vi "Read Pin.vi"(8 "error in (no error)":errorcluster, 9 "Pin 2":dbl caption="Pin", 10 "Port 4":dbl caption="Port", 11 "Arduino in":refnum<class "Arduino.lvclass">) -> (0 "error out":errorcluster, 3 "Arduino out":refnum<class "Arduino.lvclass">)   [LabVIEW 2020, in "Arduino.lvclass"]
uses:
  Arduino.lvclass
  Arduino.lvclass/Arduino.ctl
  713354a0-7d03-489a-938a-0a5a614069ab.vi
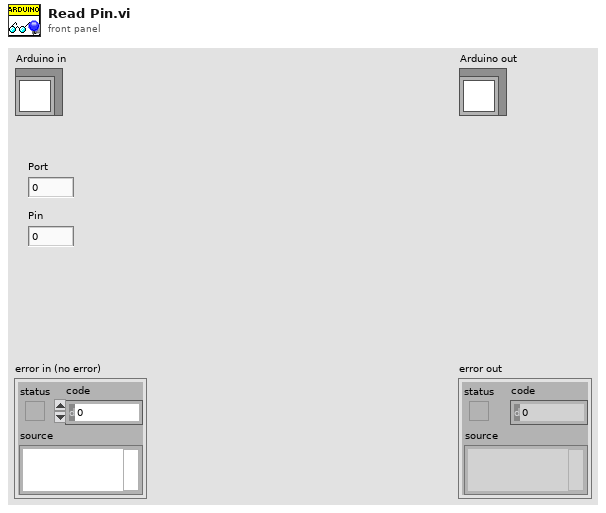
[diagram p1: front panel]
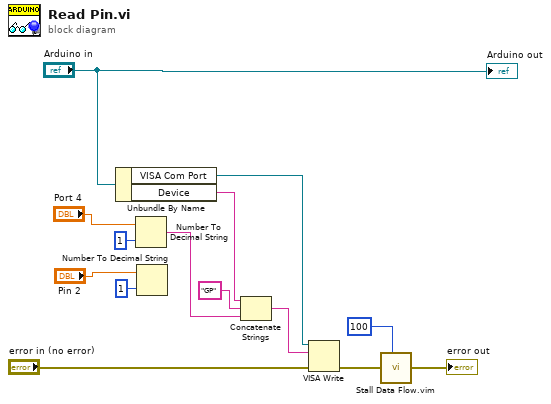
[diagram p0: block diagram]
diagram:
  n1 = Unbundle By Name("Arduino in") -> ("VISA Com Port"=w11:refnum<visa-resource-name>, "Device"=w9:string)
  n2 = Number To Decimal String(number="Port 4", width (-)=i16 1) -> (decimal integer string=w8:string)
  n3 = Number To Decimal String(number="Pin 2", width (-)=i16 1) -> ()  [unwired: 1 out]
  n4 = Concatenate Strings(w9, "GP" ("string"), w8) -> (w10:string)
  n5 = VISA Write(VISA resource name=w11, write buffer=w10) -> (error out=w12:errorcluster)  [unwired: 1 in, 2 out]
  n6 = call "Stall Data Flow.vim"("value in"=w12, "milliseconds to wait"=u32 100) -> ()  [unwired: 2 out]
  "error out" <- "error in (no error)"
  "Arduino out" <- "Arduino in"
